vi "makeScrewArray.vi"(10 "start":dbl, 11 "Cam 0":T1) -> (3 "Array":i32[][](array[numeric]))   [LabVIEW 2020, in "MagAnalysis_Online.lvclass"]
uses:
  MagAnalysis_Online.lvclass
  srew_TypDEf.ctl
  ScrewSub_Typdef.ctl
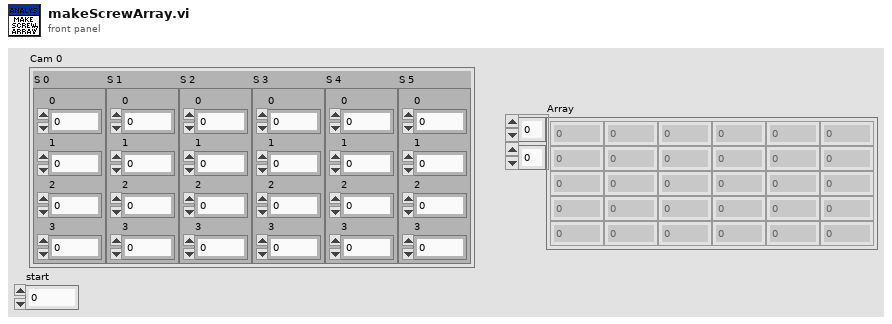
[diagram p1: front panel]
types:
  T1 = typedef "srew_TypDEf.ctl" = cluster{"S 0":T2, "S 1":T2, "S 2":T2, "S 3":T2, "S 4":T2, "S 5":T2}
  T2 = typedef "ScrewSub_Typdef.ctl" = cluster{"0":i32, "1":i32, "2":i32, "3":i32}
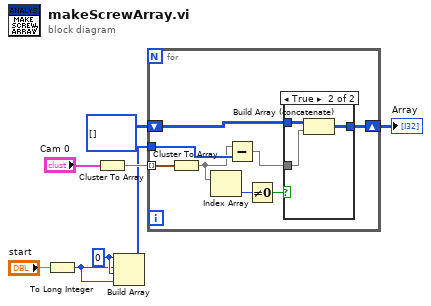
[diagram p0: block diagram]
diagram:
  w4 = 0 ("element")
  n1 = To Long Integer(number="start") -> (32bit integer=w1:i32)
  n2 = Cluster To Array(cluster="Cam 0") -> (array=w6:T2[])
  n3 = Build Array(w4, w1, w4, w1) -> (w3:i32[])
  n4 = for {
    tunnel: w6 -> [w16] mode=indexing
    shift-right: [w13] -> w8
    shift-left: i32[][] [] -> [w12]
    tunnel: w3 -> [w11]
    n5 = Cluster To Array(cluster=w16) -> (array=w10:i32[])
    n6 = Index Array(array=w10) -> (element=w15:i32)  [unwired: 1 in]
    n7 = Subtract(x=w10, y=w11) -> (x-y=w9:i32[])
    n8 = Not Equal To 0?(x=w15) -> (x != 0?=w14:bool)
    n9 = case shown="True" w14 {
      tunnel: w9 -> [_ w20]
      tunnel: [w17 w19] -> w13
      tunnel: w12 -> [w17 w18]
      frame False {
      }
      frame True {
        n10 = Build Array (concatenate)(w18, w20) -> (w19:i32[][])
      }
    }
  }
  "Array" <- w8
